vi "raedCameraAttributes.vi"(7 "error in":errorcluster) -> (20 "Image Out":T2(plugin-control), 27 "error out":errorcluster)   [LabVIEW 2020]
doc: "Creates, and edits acquisitions using the NI Vision Acquisition Express VI.\n\nThe NI Vision Acquisition Wizard is launched by placing the Express VI on the block diagram. Select an acquisition source and configure an acquisition using NI-IMAQ, NI-IMAQdx, or simulate an acquisition by reading an AVI or image files from a folder. After an acquisition is configured, select controls and indicators to be able to programmatically set in LabVIEW. Double-click the Vision Acquisition Express VI to edit the acquisition.\n\nNote: Any images created by the Express VI need to be disposed after use. Use the IMAQ Dispose.vi to cleanup the images output by the Express VI when they are no longer needed."
uses:
  <vilib>/userdefined/High Color/IMAQdx.ctl
  <vilib>/vision/driver/NI_Vision_Acquisition_Software.lvlib
panel:
  in  "Session In":T1
  out "Table Control":string[][](table)=[["AcquisitionAttributes::AdvancedGenicam::CommandTimeout", "U32", "Writable", "Readable"], ["AcquisitionAttributes::AdvancedGenicam::EventQueueDepth", "U32", "Writable", "Readable"], ["AcquisitionAttributes::AdvancedGenicam::EventsEnabled", "Bool", "Writable", "Readable"], ["AcquisitionAttributes::AdvancedGenicam::EventsSupported", "Bool", "----", "Readable"], ["AcquisitionAttributes::AdvancedGenicam::IgnoreCameraValidationErrors", "Bool", "Writable", "Readable"], ["AcquisitionAttributes::AdvancedUSB3Vision::ActualMaximumPayloadTransferSize", "U32", "----", "Readable"], ["AcquisitionAttributes::AdvancedUSB3Vision::RequiredPayloadSizeAlignment", "U32", "----", "Readable"], ["AcquisitionAttributes::Bayer::Algorithm", "Enum", "Writable", "Readable"], ["AcquisitionAttributes::Bayer::GainB", "DBL", "Writable", "Readable"], ["AcquisitionAttributes::Bayer::GainG", "DBL", "Writable", "Readable"], ["AcquisitionAttributes::Bayer::GainR", "DBL", "Writable", "Readable"], ["AcquisitionAttributes::Bayer::Pattern", "Enum", "Writable", "Readable"], ["AcquisitionAttributes::ChunkDataDecoding::ChunkDataDecodingEnabled", "Bool", "----", "Readable"], ["AcquisitionAttributes::ChunkDataDecoding::MaximumChunkCopySize", "U32", "----", "Readable"], ["CameraAttributes::AcquisitionControl::AcquisitionMode", "Enum", "----", "Readable"], ["CameraAttributes::AcquisitionControl::AcquisitionFrameCount", "I64", "----", "Readable"], ["CameraAttributes::AcquisitionControl::AcquisitionBurstFrameCount", "I64", "Writable", "Readable"], ["CameraAttributes::AcquisitionControl::ExposureMode", "Enum", "Writable", "Readable"], ["CameraAttributes::AcquisitionControl::ExposureTime", "DBL", "Writable", "Readable"], ["CameraAttributes::AcquisitionControl::ExposureAuto", "Enum", "Writable", "Readable"], ["CameraAttributes::AcquisitionControl::AcquisitionFrameRate", "DBL", "----", "Readable"], ["CameraAttributes::AcquisitionControl::AcquisitionResultingFrameRate", "DBL", "----", "Readable"], ["CameraAttributes::AcquisitionControl::AcquisitionFrameRateEnable", "Bool", "Writable", "Readable"], ["CameraAttributes::AcquisitionControl::AcquisitionLineRate", "DBL", "----", "Readable"], ["CameraAttributes::AcquisitionControl::TriggerSelector", "Enum", "Writable", "Readable"], ["CameraAttributes::AcquisitionControl::TriggerMode", "Enum", "Writable", "Readable"], ["CameraAttributes::AcquisitionControl::TriggerSoftware", "Command", "----", "----"], ["CameraAttributes::AcquisitionControl::TriggerSource", "Enum", "Writable", "Readable"], ["CameraAttributes::AcquisitionControl::TriggerActivation", "Enum", "----", "----"], ["CameraAttributes::AcquisitionControl::TriggerOverlap", "Enum", "Writable", "Readable"], ["CameraAttributes::AcquisitionControl::TriggerDelay", "DBL", "Writable", "Readable"], ["CameraAttributes::AcquisitionControl::SensorShutterMode", "Enum", "----", "Readable"], ["CameraAttributes::AnalogControl::GainSelector", "Enum", "Writable", "Readable"], ["CameraAttributes::AnalogControl::Gain", "DBL", "Writable", "Readable"], ["CameraAttributes::AnalogControl::GainAuto", "Enum", "Writable", "Readable"], ["CameraAttributes::AnalogControl::BlackLevelSelector", "Enum", "Writable", "Readable"], ["CameraAttributes::AnalogControl::BlackLevelRaw", "I64", "----", "----"], ["CameraAttributes::AnalogControl::BlackLevel", "DBL", "Writable", "Readable"], ["CameraAttributes::AnalogControl::BlackLevelClampingEnable", "Bool", "----", "Readable"], ["CameraAttributes::AnalogControl::BalanceRatioSelector", "Enum", "----", "----"], ["CameraAttributes::AnalogControl::BalanceRatio", "DBL", "----", "----"], ["CameraAttributes::AnalogControl::BalanceWhiteAuto", "Enum", "----", "----"], ["CameraAttributes::AnalogControl::Gamma", "DBL", "Writable", "Readable"], ["CameraAttributes::AnalogControl::GammaEnable", "Bool", "Writable", "Readable"], ["CameraAttributes::AnalogControl::SharpeningEnable", "Bool", "----", "----"], ["CameraAttributes::AnalogControl::SharpeningAuto", "Bool", "----", "----"], ["CameraAttributes::AnalogControl::Sharpening", "DBL", "----", "----"], ["CameraAttributes::AnalogControl::SharpeningThreshold", "DBL", "----", "----"], ["CameraAttributes::ImageFormatControl::SensorWidth", "I64", "----", "Readable"], ["CameraAttributes::ImageFormatControl::SensorHeight", "I64", "----", "Readable"], ["CameraAttributes::ImageFormatControl::WidthMax", "I64", "----", "Readable"], ["CameraAttributes::ImageFormatControl::HeightMax", "I64", "----", "Readable"], ["CameraAttributes::ImageFormatControl::Width", "I64", "----", "Readable"], ["CameraAttributes::ImageFormatControl::Height", "I64", "----", "Readable"], ["CameraAttributes::ImageFormatControl::OffsetX", "I64", "Writable", "Readable"], ["CameraAttributes::ImageFormatControl::OffsetY", "I64", "Writable", "Readable"], ["CameraAttributes::ImageFormatControl::PixelFormat", "Enum", "----", "Readable"], ["CameraAttributes::ImageFormatControl::PixelSize", "Enum", "----", "Readable"], ["CameraAttributes::ImageFormatControl::PixelColorFilter", "Enum", "----", "Readable"], ["CameraAttributes::ImageFormatControl::PixelDynamicRangeMin", "I64", "----", "Readable"], ["CameraAttributes::ImageFormatControl::PixelDynamicRangeMax", "I64", "----", "Readable"], ["CameraAttributes::ImageFormatControl::IspEnable", "Bool", "----", "Readable"], ["CameraAttributes::ImageFormatControl::BinningSelector", "Enum", "Writable", "Readable"], ["CameraAttributes::ImageFormatControl::BinningHorizontalMode", "Enum", "----", "Readable"], ["CameraAttributes::ImageFormatControl::BinningVerticalMode", "Enum", "----", "Readable"], ["CameraAttributes::ImageFormatControl::BinningHorizontal", "I64", "----", "Readable"], ["CameraAttributes::ImageFormatControl::BinningVertical", "I64", "----", "Readable"], ["CameraAttributes::ImageFormatControl::DecimationSelector", "Enum", "Writable", "Readable"], ["CameraAttributes::ImageFormatControl::DecimationHorizontalMode", "Enum", "Writable", "Readable"], ["CameraAttributes::ImageFormatControl::DecimationVerticalMode", "Enum", "Writable", "Readable"], ["CameraAttributes::ImageFormatControl::DecimationHorizontal", "I64", "----", "Readable"], ["CameraAttributes::ImageFormatControl::DecimationVertical", "I64", "----", "Readable"], ["CameraAttributes::ImageFormatControl::ReverseX", "Bool", "----", "Readable"], ["CameraAttributes::ImageFormatControl::ReverseY", "Bool", "----", "Readable"], ["CameraAttributes::ImageFormatControl::TestPatternGeneratorSelector", "Enum", "Writable", "Readable"], ["CameraAttributes::ImageFormatControl::TestPattern", "Enum", "----", "Readable"], ["CameraAttributes::ImageFormatControl::AdcBitDepth", "Enum", "----", "Readable"], ["CameraAttributes::DeviceControl::DeviceScanType", "Enum", "----", "Readable"], ["CameraAttributes::DeviceControl::DeviceVendorName", "String", "----", "Readable"], ["CameraAttributes::DeviceControl::DeviceModelName", "String", "----", "Readable"], ["CameraAttributes::DeviceControl::SensorDescription", "String", "----", "Readable"], ["CameraAttributes::DeviceControl::DeviceFirmwareVersion", "String", "----", "Readable"], ["CameraAttributes::DeviceControl::DeviceSerialNumber", "String", "----", "Readable"], ["CameraAttributes::DeviceControl::DeviceUserID", "String", "Writable", "Readable"], ["CameraAttributes::DeviceControl::DeviceTLType", "Enum", "----", "Readable"], ["CameraAttributes::DeviceControl::DeviceGenCPVersionMajor", "I64", "----", "Readable"], ["CameraAttributes::DeviceControl::DeviceGenCPVersionMinor", "I64", "----", "Readable"], ["CameraAttributes::DeviceControl::DeviceMaxThroughput", "I64", "----", "Readable"], ["CameraAttributes::DeviceControl::DeviceLinkSpeed", "I64", "----", "Readable"], ["CameraAttributes::DeviceControl::DeviceLinkThroughputLimit", "I64", "Writable", "Readable"], ["CameraAttributes::DeviceControl::DeviceLinkBandwidthReserve", "DBL", "Writable", "Readable"], ["CameraAttributes::DeviceControl::DeviceLinkCurrentThroughput", "I64", "----", "Readable"], ["CameraAttributes::DeviceControl::DeviceIndicatorMode", "Enum", "Writable", "Readable"], ["CameraAttributes::DeviceControl::DeviceTemperatureSelector", "Enum", "Writable", "Readable"], ["CameraAttributes::DeviceControl::DeviceTemperature", "DBL", "----", "Readable"], ["CameraAttributes::DeviceControl::TimestampLatch", "Command", "Writable", "----"], ["CameraAttributes::DeviceControl::TimestampLatchValue", "I64", "----", "Readable"], ["CameraAttributes::DeviceControl::TimestampIncrement", "I64", "----", "Readable"], ["CameraAttributes::DeviceControl::DevicePowerSupplySelector", "Enum", "Writable", "Readable"], ["CameraAttributes::DeviceControl::PowerSupplyVoltage", "DBL", "----", "Readable"], ["CameraAttributes::DeviceControl::PowerSupplyCurrent", "DBL", "----", "Readable"], ["CameraAttributes::DeviceControl::DeviceUptime", "I64", "----", "Readable"], ["CameraAttributes::DeviceControl::LinkUptime", "I64", "----", "Readable"], ["CameraAttributes::DeviceControl::EnumerationCount", "I64", "----", "Readable"], ["CameraAttributes::DeviceControl::FactoryReset", "Command", "Writable", "----"], ["CameraAttributes::DeviceControl::MaxDeviceResetTime", "I64", "----", "Readable"], ["CameraAttributes::TransportLayerControl::PayloadSize", "I64", "----", "Readable"], ["CameraAttributes::TransportLayerControl::USB3Vision::U3VMessageChannelID", "I64", "Writable", "Readable"], ["CameraAttributes::TransportLayerControl::USB3Vision::U3VVersionMajor", "I64", "----", "Readable"], ["CameraAttributes::TransportLayerControl::USB3Vision::U3VVersionMinor", "I64", "----", "Readable"], ["CameraAttributes::TransportLayerControl::USB3Vision::U3VCPCapability", "I64", "----", "Readable"], ["CameraAttributes::TransportLayerControl::USB3Vision::U3VCPSIRMAvailable", "Bool", "----", "Readable"], ["CameraAttributes::TransportLayerControl::USB3Vision::U3VCPEIRMAvailable", "Bool", "----", "Readable"], ["CameraAttributes::TransportLayerControl::USB3Vision::U3VCPIIDC2Available", "Bool", "----", "Readable"], ["CameraAttributes::TransportLayerControl::USB3Vision::U3VMaxCommandTransferLength", "I64", "----", "Readable"], ["CameraAttributes::TransportLayerControl::USB3Vision::U3VMaxAcknowledgeTransferLength", "I64", "----", "Readable"], ["CameraAttributes::TransportLayerControl::USB3Vision::U3VNumberOfStreamChannels", "I64", "----", "Readable"], ["CameraAttributes::TransportLayerControl::USB3Vision::U3VCurrentSpeed", "Enum", "----", "Readable"], ["CameraAttributes::TransportLayerControl::LinkErrorCount", "I64", "----", "Readable"], ["CameraAttributes::TransportLayerControl::LinkRecoveryCount", "I64", "----", "Readable"], ["CameraAttributes::SequencerControl::SequencerMode", "Enum", "----", "Readable"], ["CameraAttributes::SequencerControl::SequencerConfigurationMode", "Enum", "Writable", "Readable"], ["CameraAttributes::SequencerControl::SequencerConfigurationValid", "Enum", "----", "Readable"], ["CameraAttributes::SequencerControl::SequencerConfigurationReset", "Command", "----", "----"], ["CameraAttributes::SequencerControl::SequencerFeatureSelector", "Enum", "Writable", "Readable"], ["CameraAttributes::SequencerControl::SequencerFeatureEnable", "Bool", "Writable", "Readable"], ["CameraAttributes::SequencerControl::SequencerSetStart", "I64", "----", "Readable"], ["CameraAttributes::SequencerControl::SequencerSetActive", "I64", "----", "----"], ["CameraAttributes::SequencerControl::SequencerSetSelector", "I64", "Writable", "Readable"], ["CameraAttributes::SequencerControl::SequencerSetValid", "Enum", "----", "Readable"], ["CameraAttributes::SequencerControl::SequencerSetSave", "Command", "----", "----"], ["CameraAttributes::SequencerControl::SequencerSetLoad", "Command", "----", "----"], ["CameraAttributes::SequencerControl::SequencerPathSelector", "I64", "Writable", "Readable"], ["CameraAttributes::SequencerControl::SequencerTriggerSource", "Enum", "----", "Readable"], ["CameraAttributes::SequencerControl::SequencerTriggerActivation", "Enum", "----", "----"], ["CameraAttributes::SequencerControl::SequencerSetNext", "I64", "----", "----"], ["CameraAttributes::ColorTransformationControl::ColorTransformationSelector", "Enum", "----", "----"], ["CameraAttributes::ColorTransformationControl::ColorTransformationEnable", "Bool", "----", "----"], ["CameraAttributes::ColorTransformationControl::ColorTransformationValueSelector", "Enum", "----", "----"], ["CameraAttributes::ColorTransformationControl::ColorTransformationValue", "DBL", "----", "----"], ["CameraAttributes::ColorTransformationControl::RgbTransformLightSource", "Enum", "----", "----"], ["CameraAttributes::ColorTransformationControl::SaturationEnable", "Bool", "----", "----"], ["CameraAttributes::ColorTransformationControl::Saturation", "DBL", "----", "----"], ["CameraAttributes::AutoAlgorithmControl::AutoAlgorithmSelector", "Enum", "Writable", "Readable"], ["CameraAttributes::AutoAlgorithmControl::AasRoiEnable", "Bool", "----", "----"], ["CameraAttributes::AutoAlgorithmControl::AasRoiOffsetX", "I64", "----", "----"], ["CameraAttributes::AutoAlgorithmControl::AasRoiOffsetY", "I64", "----", "----"], ["CameraAttributes::AutoAlgorithmControl::AasRoiWidth", "I64", "----", "----"], ["CameraAttributes::AutoAlgorithmControl::AasRoiHeight", "I64", "----", "----"], ["CameraAttributes::AutoAlgorithmControl::BalanceWhiteAutoProfile", "Enum", "----", "----"], ["CameraAttributes::AutoAlgorithmControl::BalanceWhiteAutoLowerLimit", "DBL", "----", "----"], ["CameraAttributes::AutoAlgorithmControl::BalanceWhiteAutoUpperLimit", "DBL", "----", "----"], ["CameraAttributes::AutoAlgorithmControl::BalanceWhiteAutoDamping", "DBL", "----", "----"], ["CameraAttributes::AutoAlgorithmControl::AutoExposureTargetGreyValueAuto", "Enum", "Writable", "Readable"], ["CameraAttributes::AutoAlgorithmControl::AutoExposureTargetGreyValue", "DBL", "----", "----"], ["CameraAttributes::AutoAlgorithmControl::AutoExposureLightingMode", "Enum", "Writable", "Readable"], ["CameraAttributes::AutoAlgorithmControl::AutoExposureMeteringMode", "Enum", "Writable", "Readable"], ["CameraAttributes::AutoAlgorithmControl::AutoExposureExposureTimeLowerLimit", "DBL", "Writable", "Readable"], ["CameraAttributes::AutoAlgorithmControl::AutoExposureExposureTimeUpperLimit", "DBL", "Writable", "Readable"], ["CameraAttributes::AutoAlgorithmControl::AutoExposureGainLowerLimit", "DBL", "Writable", "Readable"], ["CameraAttributes::AutoAlgorithmControl::AutoExposureGainUpperLimit", "DBL", "Writable", "Readable"], ["CameraAttributes::AutoAlgorithmControl::AutoExposureGreyValueLowerLimit", "DBL", "Writable", "Readable"], ["CameraAttributes::AutoAlgorithmControl::AutoExposureGreyValueUpperLimit", "DBL", "Writable", "Readable"], ["CameraAttributes::AutoAlgorithmControl::AutoExposureEVCompensation", "DBL", "Writable", "Readable"], ["CameraAttributes::AutoAlgorithmControl::AutoExposureControlLoopDamping", "DBL", "Writable", "Readable"], ["CameraAttributes::AutoAlgorithmControl::AutoExposureControlPriority", "Enum", "----", "----"], ["CameraAttributes::FlatFieldCorrectionControl::FfcEnable", "Bool", "----", "----"], ["CameraAttributes::FlatFieldCorrectionControl::FfcMode", "Enum", "----", "----"], ["CameraAttributes::FlatFieldCorrectionControl::FfcUserTableControl::FfcUserTableXCoordinate", "I64", "----", "----"], ["CameraAttributes::FlatFieldCorrectionControl::FfcUserTableControl::FfcUserGain", "DBL", "----", "----"], ["CameraAttributes::FlatFieldCorrectionControl::FfcUserTableControl::FfcUserOffset", "I64", "----", "----"], ["CameraAttributes::FlatFieldCorrectionControl::FfcUserTableControl::FfcUserTableReset", "Command", "----", "----"], ["CameraAttributes::FlatFieldCorrectionControl::FfcUserTableControl::FfcUserTableSave", "Command", "----", "----"], ["CameraAttributes::DefectivePixelCorrection::DefectCorrectStaticEnable", "Bool", "Writable", "Readable"], ["CameraAttributes::DefectivePixelCorrection::DefectCorrectionMode", "Enum", "Writable", "Readable"], ["CameraAttributes::DefectivePixelCorrection::DefectTablePixelCount", "I64", "Writable", "Readable"], ["CameraAttributes::DefectivePixelCorrection::DefectTableIndex", "I64", "Writable", "Readable"], ["CameraAttributes::DefectivePixelCorrection::DefectTableCoordinateX", "I64", "Writable", "Readable"], ["CameraAttributes::DefectivePixelCorrection::DefectTableCoordinateY", "I64", "Writable", "Readable"], ["CameraAttributes::DefectivePixelCorrection::DefectTableApply", "Command", "----", "----"], ["CameraAttributes::DefectivePixelCorrection::DefectTableSave", "Command", "----", "----"], ["CameraAttributes::DefectivePixelCorrection::DefectTableFactoryRestore", "Command", "----", "----"], ["CameraAttributes::UserSetControl::UserSetSelector", "Enum", "Writable", "Readable"], ["CameraAttributes::UserSetControl::UserSetLoad", "Command", "----", "----"], ["CameraAttributes::UserSetControl::UserSetSave", "Command", "----", "----"], ["CameraAttributes::UserSetControl::UserSetDefault", "Enum", "Writable", "Readable"], ["CameraAttributes::UserSetControl::UserSetFeatureSelector", "Enum", "Writable", "Readable"], ["CameraAttributes::UserSetControl::UserSetFeatureEnable", "Bool", "----", "Readable"], ["CameraAttributes::ChunkDataControl::ChunkModeActive", "Bool", "----", "Readable"], ["CameraAttributes::ChunkDataControl::ChunkSelector", "Enum", "Writable", "Readable"], ["CameraAttributes::ChunkDataControl::ChunkEnable", "Bool", "----", "Readable"], ["CameraAttributes::ChunkDataControl::ChunkImage", "I64", "----", "----"], ["CameraAttributes::ChunkDataControl::ChunkCRC", "I64", "----", "----"], ["CameraAttributes::ChunkDataControl::ChunkFrameID", "I64", "----", "----"], ["CameraAttributes::ChunkDataControl::ChunkOffsetX", "I64", "----", "----"], ["CameraAttributes::ChunkDataControl::ChunkOffsetY", "I64", "----", "----"], ["CameraAttributes::ChunkDataControl::ChunkWidth", "I64", "----", "----"], ["CameraAttributes::ChunkDataControl::ChunkHeight", "I64", "----", "----"], ["CameraAttributes::ChunkDataControl::ChunkPixelFormat", "Enum", "----", "----"], ["CameraAttributes::ChunkDataControl::ChunkExposureTime", "DBL", "----", "----"], ["CameraAttributes::ChunkDataControl::ChunkGainSelector", "Enum", "Writable", "Readable"], ["CameraAttributes::ChunkDataControl::ChunkGain", "DBL", "----", "----"], ["CameraAttributes::ChunkDataControl::ChunkBlackLevelSelector", "Enum", "Writable", "Readable"], ["CameraAttributes::ChunkDataControl::ChunkBlackLevel", "DBL", "----", "----"], ["CameraAttributes::ChunkDataControl::ChunkTimestamp", "I64", "----", "----"], ["CameraAttributes::ChunkDataControl::ChunkSequencerSetActive", "I64", "----", "----"], ["CameraAttributes::ChunkDataControl::ChunkSerialDataLength", "I64", "----", "----"], ["CameraAttributes::ChunkDataControl::ChunkSerialData", "String", "----", "----"], ["CameraAttributes::ChunkDataControl::ChunkSerialReceiveOverflow", "Bool", "----", "----"], ["CameraAttributes::LUTControl::LUTSelector", "Enum", "Writable", "Readable"], ["CameraAttributes::LUTControl::LUTEnable", "Bool", "Writable", "Readable"], ["CameraAttributes::LUTControl::LUTIndex", "I64", "Writable", "Readable"], ["CameraAttributes::LUTControl::LUTValue", "I64", "Writable", "Readable"], ["CameraAttributes::EventControl::EventSelector", "Enum", "Writable", "Readable"], ["CameraAttributes::EventControl::EventNotification", "Enum", "Writable", "Readable"], ["CameraAttributes::EventControl::EventExposureEndData::EventExposureEnd", "I64", "----", "Readable"], ["CameraAttributes::EventControl::EventExposureEndData::EventExposureEndTimestamp", "I64", "----", "----"], ["CameraAttributes::EventControl::EventExposureEndData::EventExposureEndFrameID", "I64", "----", "----"], ["CameraAttributes::EventControl::EventErrorData::EventError", "I64", "----", "Readable"], ["CameraAttributes::EventControl::EventErrorData::EventErrorTimestamp", "I64", "----", "----"], ["CameraAttributes::EventControl::EventErrorData::EventErrorFrameID", "I64", "----", "----"], ["CameraAttributes::EventControl::EventErrorData::EventErrorCode", "I64", "----", "----"], ["CameraAttributes::EventControl::EventSerialPortReceiveData::EventSerialPortReceive", "I64", "----", "Readable"], ["CameraAttributes::EventControl::EventSerialPortReceiveData::EventSerialPortReceiveTimestamp", "I64", "----", "----"], ["CameraAttributes::EventControl::EventSerialPortReceiveData::EventSerialData", "String", "----", "----"], ["CameraAttributes::EventControl::EventSerialPortReceiveData::EventSerialDataLength", "I64", "----", "----"], ["CameraAttributes::EventControl::EventSerialPortReceiveData::EventSerialReceiveOverflow", "Bool", "----", "----"], ["CameraAttributes::EventControl::EventTestData::EventTest", "I64", "----", "Readable"], ["CameraAttributes::EventControl::EventTestData::EventTestTimestamp", "I64", "----", "----"], ["CameraAttributes::CounterAndTimerControl::CounterSelector", "Enum", "Writable", "Readable"], ["CameraAttributes::CounterAndTimerControl::CounterEventSource", "Enum", "Writable", "Readable"], ["CameraAttributes::CounterAndTimerControl::CounterEventActivation", "Enum", "----", "----"], ["CameraAttributes::CounterAndTimerControl::CounterDuration", "I64", "Writable", "Readable"], ["CameraAttributes::CounterAndTimerControl::CounterValue", "I64", "----", "Readable"], ["CameraAttributes::CounterAndTimerControl::CounterValueAtReset", "I64", "----", "----"], ["CameraAttributes::CounterAndTimerControl::CounterTriggerSource", "Enum", "Writable", "Readable"], ["CameraAttributes::CounterAndTimerControl::CounterTriggerActivation", "Enum", "Writable", "Readable"], ["CameraAttributes::CounterAndTimerControl::CounterResetSource", "Enum", "----", "----"], ["CameraAttributes::CounterAndTimerControl::CounterResetActivation", "Enum", "----", "----"], ["CameraAttributes::CounterAndTimerControl::CounterStatus", "Enum", "----", "Readable"], ["CameraAttributes::CounterAndTimerControl::CounterDelay", "I64", "Writable", "Readable"], ["CameraAttributes::TestControl::TestPendingAck", "I64", "Writable", "Readable"], ["CameraAttributes::TestControl::TestEventGenerate", "Command", "Writable", "----"], ["CameraAttributes::TestControl::Test0001", "I64", "Writable", "Readable"], ["CameraAttributes::LogicBlockControl::LogicBlockSelector", "Enum", "Writable", "Readable"], ["CameraAttributes::LogicBlockControl::LogicBlockLUTSelector", "Enum", "Writable", "Readable"], ["CameraAttributes::LogicBlockControl::LogicBlockLUTInputSelector", "Enum", "Writable", "Readable"], ["CameraAttributes::LogicBlockControl::LogicBlockLUTInputSource", "Enum", "Writable", "Readable"], ["CameraAttributes::LogicBlockControl::LogicBlockLUTInputActivation", "Enum", "Writable", "Readable"], ["CameraAttributes::LogicBlockControl::LogicBlockLUTOutputValueAll", "I64", "Writable", "Readable"], ["CameraAttributes::LogicBlockControl::LogicBlockLUTRowIndex", "I64", "Writable", "Readable"], ["CameraAttributes::LogicBlockControl::LogicBlockLUTOutputValue", "Bool", "Writable", "Readable"], ["CameraAttributes::DigitalIOControl::LineSelector", "Enum", "Writable", "Readable"], ["CameraAttributes::DigitalIOControl::LineMode", "Enum", "Writable", "Readable"], ["CameraAttributes::DigitalIOControl::V3_3Enable", "Bool", "----", "----"], ["CameraAttributes::DigitalIOControl::LineInverter", "Bool", "Writable", "Readable"], ["CameraAttributes::DigitalIOControl::LineStatus", "Bool", "----", "Readable"], ["CameraAttributes::DigitalIOControl::LineStatusAll", "I64", "----", "Readable"], ["CameraAttributes::DigitalIOControl::LineInputFilterSelector", "Enum", "Writable", "Readable"], ["CameraAttributes::DigitalIOControl::LineFilterWidth", "DBL", "Writable", "Readable"], ["CameraAttributes::DigitalIOControl::LineSource", "Enum", "Writable", "Readable"], ["CameraAttributes::DigitalIOControl::LineFormat", "Enum", "----", "Readable"], ["CameraAttributes::DigitalIOControl::UserOutputSelector", "Enum", "Writable", "Readable"], ["CameraAttributes::DigitalIOControl::UserOutputValue", "Bool", "Writable", "Readable"], ["CameraAttributes::DigitalIOControl::UserOutputValueAll", "I64", "Writable", "Readable"], ["CameraAttributes::SerialPortControl::SerialPortSelector", "Enum", "Writable", "Readable"], ["CameraAttributes::SerialPortControl::SerialPortSource", "Enum", "Writable", "Readable"], ["CameraAttributes::SerialPortControl::SerialPortBaudRate", "Enum", "Writable", "Readable"], ["CameraAttributes::SerialPortControl::SerialPortDataBits", "I64", "Writable", "Readable"], ["CameraAttributes::SerialPortControl::SerialPortStopBits", "Enum", "Writable", "Readable"], ["CameraAttributes::SerialPortControl::SerialPortParity", "Enum", "Writable", "Readable"], ["CameraAttributes::SerialPortControl::SerialTransmitQueueMaxCharacterCount", "I64", "----", "Readable"], ["CameraAttributes::SerialPortControl::SerialTransmitQueueCurrentCharacterCount", "I64", "----", "Readable"], ["CameraAttributes::SerialPortControl::SerialReceiveQueueMaxCharacterCount", "I64", "----", "Readable"], ["CameraAttributes::SerialPortControl::SerialReceiveQueueCurrentCharacterCount", "I64", "----", "Readable"], ["CameraAttributes::SerialPortControl::SerialReceiveQueueClear", "Command", "Writable", "----"], ["CameraAttributes::SerialPortControl::SerialReceiveFramingErrorCount", "I64", "----", "Readable"], ["CameraAttributes::SerialPortControl::SerialReceiveParityErrorCount", "I64", "----", "Readable"], ["CameraAttributes::FileAccessControl::FileSelector", "Enum", "Writable", "Readable"], ["CameraAttributes::FileAccessControl::FileOperationSelector", "Enum", "Writable", "Readable"], ["CameraAttributes::FileAccessControl::FileOperationExecute", "Command", "----", "----"], ["CameraAttributes::FileAccessControl::FileOpenMode", "Enum", "Writable", "Readable"], ["CameraAttributes::FileAccessControl::FileAccessOffset", "I64", "Writable", "Readable"], ["CameraAttributes::FileAccessControl::FileAccessLength", "I64", "Writable", "Readable"], ["CameraAttributes::FileAccessControl::FileOperationStatus", "Enum", "----", "Readable"], ["CameraAttributes::FileAccessControl::FileOperationResult", "I64", "----", "Readable"], ["CameraAttributes::FileAccessControl::FileSize", "I64", "----", "Readable"], ["CameraAttributes::TransferControl::TransferControlMode", "Enum", "Writable", "Readable"], ["CameraAttributes::TransferControl::TransferOperationMode", "Enum", "----", "----"], ["CameraAttributes::TransferControl::TransferBlockCount", "I64", "----", "----"], ["CameraAttributes::TransferControl::TransferQueueMaxBlockCount", "I64", "----", "Readable"], ["CameraAttributes::TransferControl::TransferQueueCurrentBlockCount", "I64", "----", "Readable"], ["CameraAttributes::TransferControl::TransferQueueOverflowCount", "I64", "----", "Readable"], ["CameraAttributes::TransferControl::TransferQueueMode", "Enum", "----", "----"], ["CameraAttributes::TransferControl::TransferStart", "Command", "----", "----"], ["CameraAttributes::TransferControl::TransferStop", "Command", "----", "----"], ["AcquisitionAttributes::BitsPerPixel", "Enum", "----", "Readable"], ["AcquisitionAttributes::HardwareMaximumQueuedBufferCount", "U32", "----", "Readable"], ["AcquisitionAttributes::HardwareRequeueBufferListThreshold", "DBL", "----", "Readable"], ["AcquisitionAttributes::ImageDecoderCopyMode", "Enum", "----", "Readable"], ["AcquisitionAttributes::IncompleteBufferMode", "Enum", "----", "Readable"], ["AcquisitionAttributes::OutputImageType", "Enum", "----", "Readable"], ["AcquisitionAttributes::OverwriteMode", "Enum", "----", "Readable"], ["AcquisitionAttributes::ReceiveTimestampMode", "Enum", "----", "Readable"], ["AcquisitionAttributes::ShiftPixelBits", "Bool", "----", "Readable"], ["AcquisitionAttributes::SwapPixelBytes", "Bool", "----", "Readable"], ["AcquisitionAttributes::Timeout", "U32", "----", "Readable"], ["CameraInformation::BaseAddress", "U32", "----", "Readable"], ["CameraInformation::BusType", "Enum", "----", "Readable"], ["CameraInformation::ModelName", "String", "----", "Readable"], ["CameraInformation::PrimaryURLString", "String", "----", "Readable"], ["CameraInformation::SecondaryURLString", "String", "----", "Readable"], ["CameraInformation::SerialNumberHigh", "U32", "----", "Readable"], ["CameraInformation::SerialNumberLow", "U32", "----", "Readable"], ["CameraInformation::USBConnectionSpeed", "Enum", "----", "Readable"], ["CameraInformation::VendorName", "String", "----", "Readable"], ["StatusInformation::AcqInProgress", "Bool", "----", "Readable"], ["StatusInformation::HandledEventCount", "I64", "----", "Readable"], ["StatusInformation::IncompleteBufferCount", "I64", "----", "Readable"], ["StatusInformation::LastBufferCount", "I64", "----", "Readable"], ["StatusInformation::LastBufferNumber", "U32", "----", "Readable"], ["StatusInformation::LostBufferCount", "I64", "----", "Readable"], ["StatusInformation::LostEventCount", "I64", "----", "Readable"]]
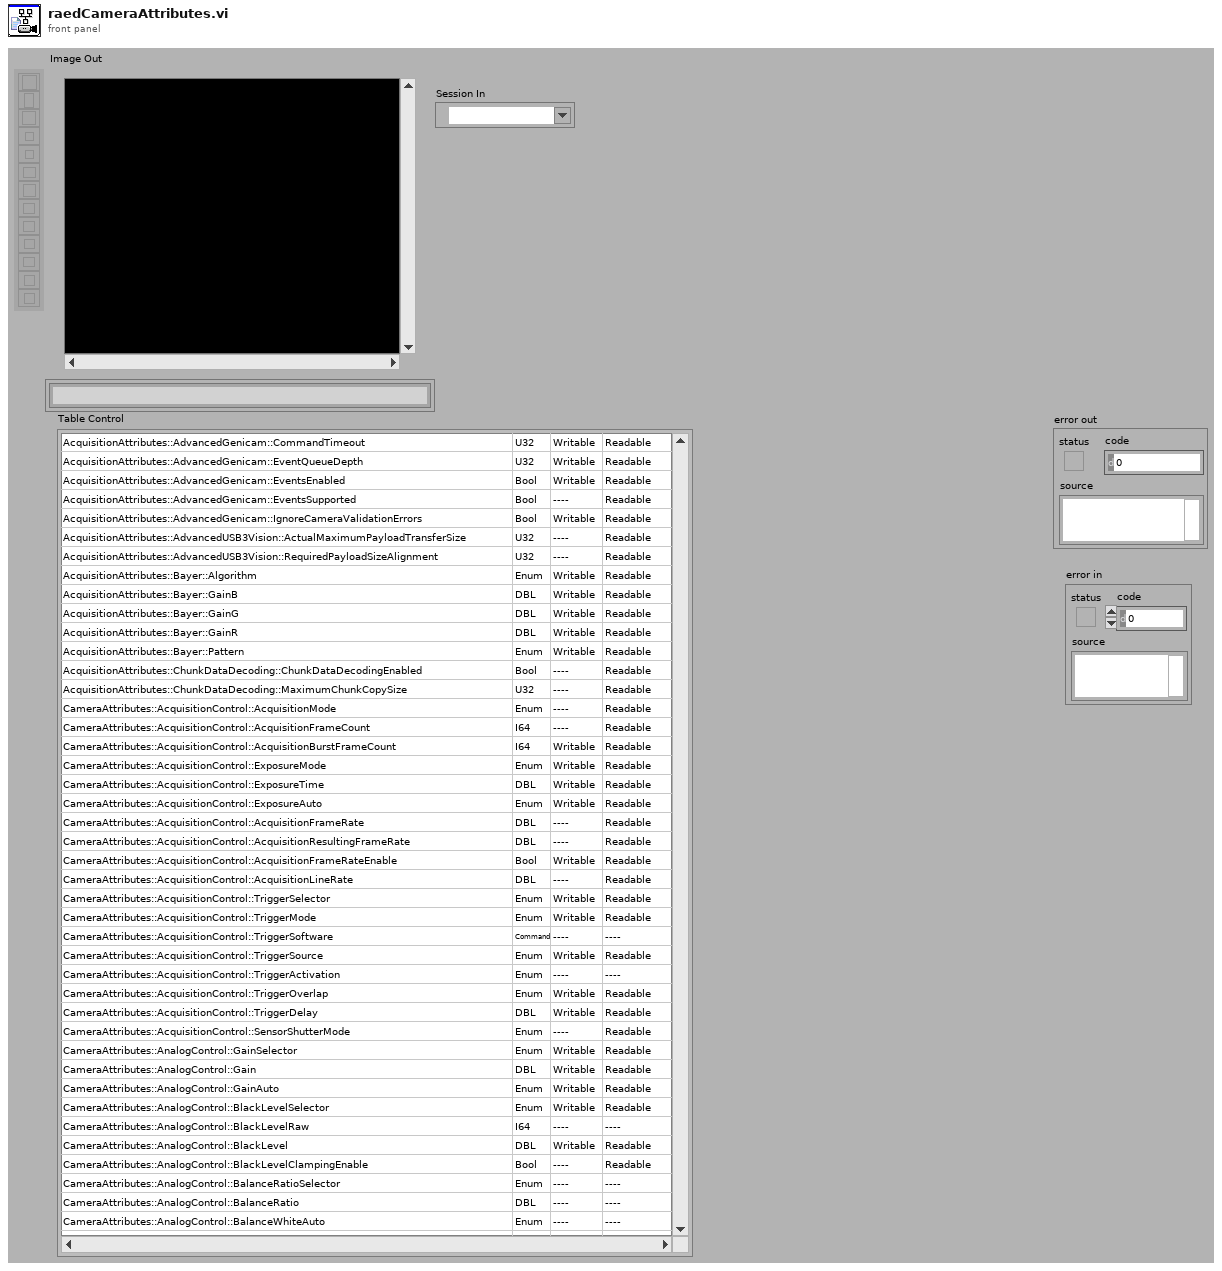
[diagram p1: front panel]
types:
  T1 = typedef "IMAQdx.ctl" = refnum<k21>
  T2 = typedef "IMAQ Image.ctl" = refnum<image>
  T3 = typedef "NI_Vision_Acquisition_Software.lvlib/IMAQdx Attribute Type.ctl" = enum32{"U32", "I64", "DBL", "String", "Enum", "Bool", "Command"}
  T4 = cluster{"Attribute Type":T3, "Readable":bool, "Writable":bool, "Attribute Name":string}[]
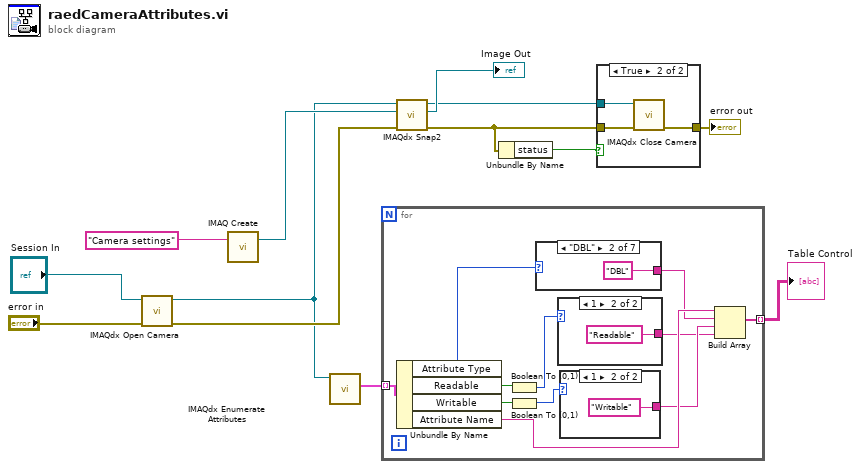
[diagram p0: block diagram]
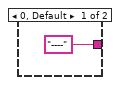
[diagram p2: hidden frame]
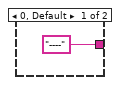
[diagram p3: hidden frame]
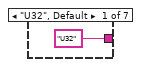
[diagram p4: hidden frame]
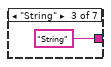
[diagram p5: hidden frame]
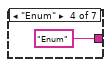
[diagram p6: hidden frame]
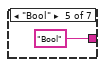
[diagram p7: hidden frame]
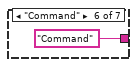
[diagram p8: hidden frame]
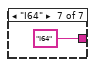
[diagram p9: hidden frame]
diagram:
  n1 = call <vilib>:"IMAQdx Open Camera.vi"("error in"="error in", "Session In"="Session In") -> ("error out"=w12:errorcluster, "Session Out"=w4:T1)  [unwired: 1 in, 7 out]
  n2 = call "IMAQ Create"("Image Name"="Camera settings") -> ("New Image"=w5:T2)  [unwired: 3 in, 2 out]
  n3 = call <vilib>:"IMAQdx Enumerate Attributes.vi"("Session In"=w4) -> ("Attribute Information Array"=w1:T4)  [unwired: 8 in, 2 out]
  n4 = for {
    tunnel: w1 -> [w14] mode=indexing
    tunnel: [w16] -> w7 mode=indexing
    n5 = Unbundle By Name(w14) -> ("Attribute Type"=w22:T3, "Readable"=w23:bool, "Writable"=w24:bool, "Attribute Name"=w19:string)
    n6 = Boolean To (0,1)(Boolean=w23) -> (0, 1=w21:i16)
    n7 = Boolean To (0,1)(Boolean=w24) -> (0, 1=w20:i16)
    n8 = case shown="\"DBL\"" w22 {
      tunnel: ["U32" "DBL" "String" "Enum" "Bool" "Command" "I64"] -> w15
      frame "U32", Default {
      }
      frame "DBL" {
      }
      frame "String" {
      }
      frame "Enum" {
      }
      frame "Bool" {
      }
      frame "Command" {
      }
      frame "I64" {
      }
    }
    n9 = case shown="1" w21 {
      tunnel: ["----" "Readable"] -> w17
      frame 0, Default {
      }
      frame 1 {
      }
    }
    n10 = case shown="1" w20 {
      tunnel: ["----" "Writable"] -> w18
      frame 0, Default {
      }
      frame 1 {
      }
    }
    n11 = Build Array(w19, w15, w18, w17) -> (w16:string[])
  }
  "Table Control" <- w7
  n12 = call <vilib>:"IMAQdx Snap2.vi"("error in"=w12, "Image In"=w5, "Session In"=w4) -> ("error out"=w10:errorcluster, "Image Out"=→"Image Out":T2, "Session Out"=w9:T1)  [unwired: 6 in]
  n13 = Unbundle By Name(w10) -> ("status"=w3:bool)
  n14 = case "Case Structure_template1" shown="True" w3 {
    tunnel: [w36 w38] -> w8
    tunnel: w10 -> [w36 w39]
    tunnel: w9 -> [_ w37]
    frame False {
    }
    frame True {
      n15 = call <vilib>:"IMAQdx Close Camera.vi"("error in"=w39, "Session In"=w37) -> ("error out"=w38:errorcluster)  [unwired: 9 out]
    }
  }
  "error out" <- w8
